vi "PID.vi"(1 "Present Value":dbl=15.0 format="%.2f", 2 "Previous Scan Value":dbl format="%.2f", 3 "Setpoint":dbl=15.0 format="%.2f") -> (0 "Dem Output":dbl format="%.2f")   [LabVIEW 2013]
uses:
  <vilib>/Analysis/NI_AALPro.lvlib
panel:
  in  "O/P deadband":dbl=1.0 format="%.2f"
  in  "Kp Deadband":dbl format="%.2f"
  in  "Derivative History":i32=20
  out "deadbanded error":dbl format="%.2f"
  in  "P":bool=TRUE
  in  "D":bool=TRUE
  in  "I":bool=TRUE
  out "Waveform Chart":T1(graph)
  in  "Manual Demand":dbl min=0.0 max=100.0 format="%.2f"
  in  "Manual Override":bool
  out "Control Sum":dbl format="%.2f"
  out "Derivative Term":dbl format="%.2f"
  out "Integral Term":dbl format="%.2f"
  out "error differential":dbl format="%.5f"
  out "error integral":dbl format="%.2f"
  out "Proportional Term":dbl format="%.2f"
  in  "Kd":dbl=25.0 format="%.2f"
  in  "Ki":dbl=0.03 format="%.3f"
  in  "Kp":dbl=1.5 format="%.2f"
  out "error":dbl format="%.2f"
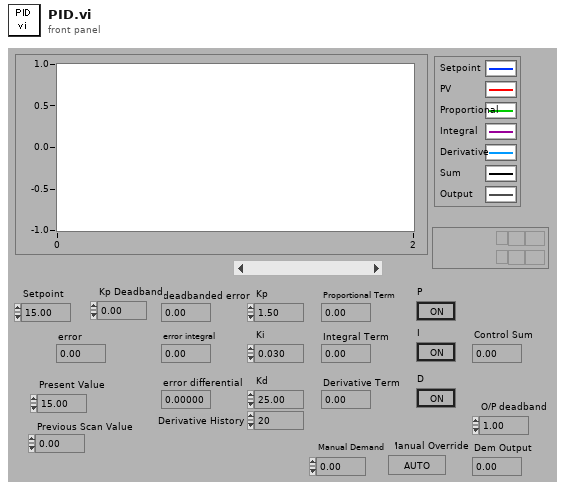
[diagram p1: front panel]
types:
  T1 = cluster{"Setpoint":dbl, "Present Value":dbl, "Proportional Term":dbl, "Integral Term":dbl, "Derivative Term":dbl, "Control Sum":dbl, "Dem Output":dbl}
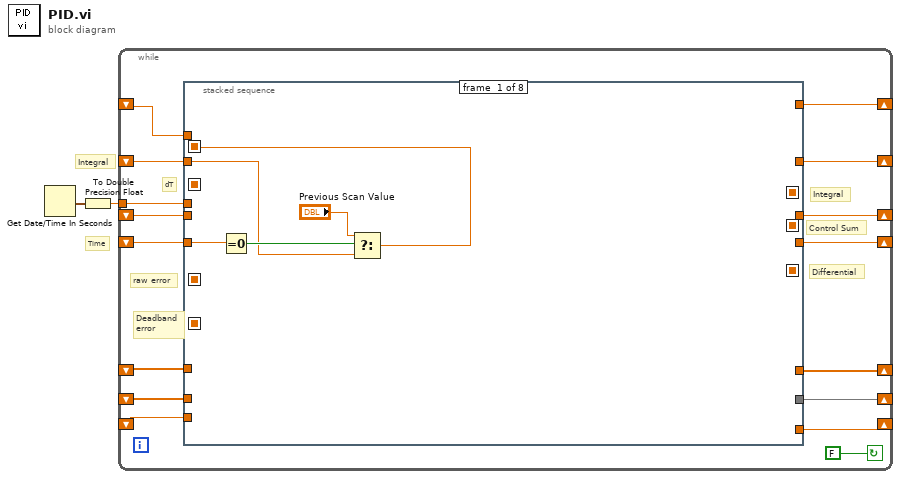
[diagram p0: block diagram]
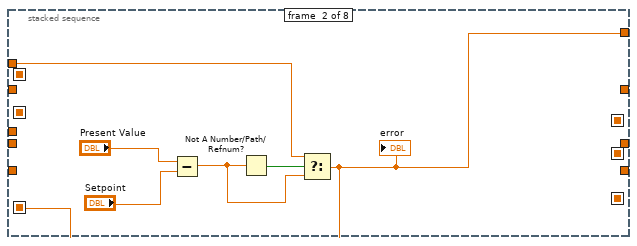
[diagram p2: hidden frame]
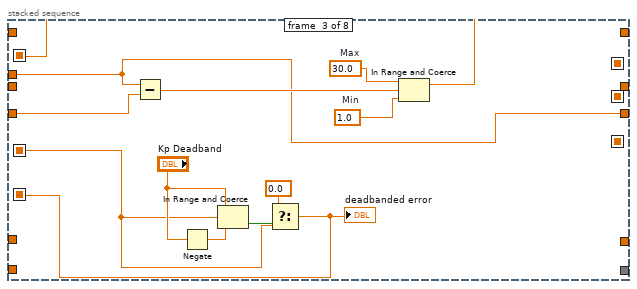
[diagram p3: hidden frame]
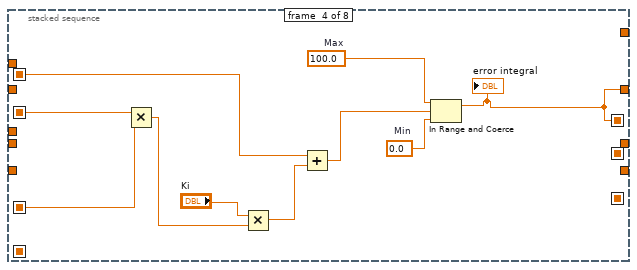
[diagram p4: hidden frame]
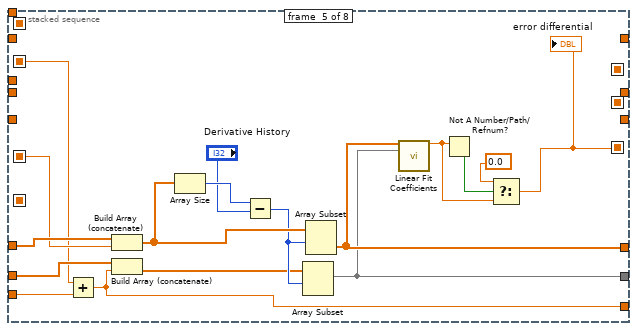
[diagram p5: hidden frame]
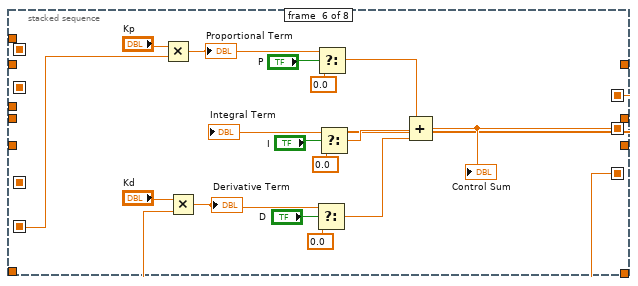
[diagram p6: hidden frame]
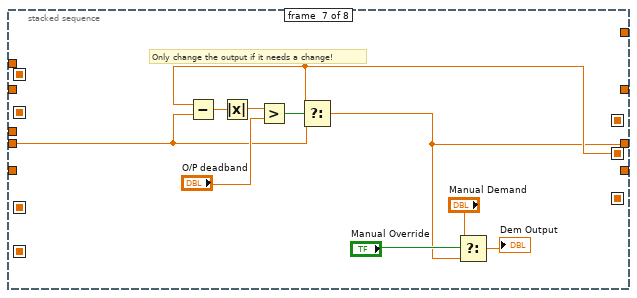
[diagram p7: hidden frame]
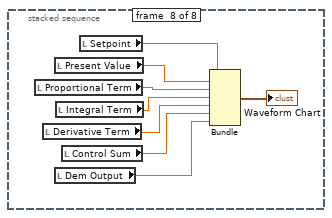
[diagram p8: hidden frame]
diagram:
  # "Integral"
  # "Time"
  n1 = Get Date/Time In Seconds() -> (seconds since 1Jan1904=w1:timestamp)
  n2 = To Double Precision Float(number=w1) -> (double precision float=w2:dbl)
  n3 = while {
    shift-left: _ -> [w5]
    shift-right: [w4] -> _
    shift-left: _ -> [w7]
    shift-right: [w6] -> _
    shift-left: _ -> [w9]
    shift-right: [w8] -> _
    tunnel: w2 -> [w14]
    shift-left: _ -> [w11]
    shift-right: [w10] -> _
    shift-left: _ -> [w13]
    shift-right: [w12] -> _
    shift-left: _ -> [w15]
    shift-right: [w16] -> _
    shift-left: _ -> [w18]
    shift-right: [w17] -> _
    stop <- FALSE continue-if-true
    # "Control Sum"
    # "raw error"
    # "Differential"
    # "Integral"
    # "Deadband\nerror"
    # "dT"
    n4 = stacked-sequence {
      seq-local: [_ _ w30 _ _ _ _ _] -> [_ _ _ w51 w54 _ _ _]
      seq-local: [_ _ w39 _ _ _ _ _] -> [_ _ _ _ _ w71 _ _]
      seq-local: [_ _ _ _ w59 _ _ _] -> [_ _ _ _ _ w70 _ _]
      seq-local: [_ _ _ w46 _ _ _ _] -> [_ _ _ _ _ w69 _ _]
      seq-local: [_ w24 _ _ _ _ _ _] -> [_ _ w31 w48 w60 _ _ _]
      seq-local: [_ _ _ _ _ w74 _ _] -> [_ _ _ _ _ _ w89 _]
      seq-local: [w19 _ _ _ _ _ _ _] -> [_ _ _ w42 _ _ _ _]
      tunnel: w18 -> [w23 _ w36 _ _ _ _ _]
      tunnel: [_ _ w34 _ _ _ _ _] -> w17
      tunnel: [_ _ _ w46 _ _ _ _] -> w16
      tunnel: w15 -> [w20 _ _ _ _ _ _ _]
      tunnel: w14 -> [_ _ w34 _ _ _ _ _]
      tunnel: w13 -> [_ _ _ _ w68 _ _ _]
      tunnel: [_ _ _ _ w61 _ _ _] -> w12
      tunnel: w11 -> [_ _ _ _ w67 _ _ _]
      tunnel: [_ _ _ _ w58 _ _ _] -> w10
      tunnel: w9 -> [_ _ _ _ _ _ w87 _]
      tunnel: [_ _ _ _ _ _ w86 _] -> w8
      tunnel: w7 -> [_ _ _ _ w53 _ _ _]
      tunnel: [_ _ _ _ w52 _ _ _] -> w6
      tunnel: w5 -> [_ w26 _ _ _ _ _ _]
      tunnel: [_ w24 _ _ _ _ _ _] -> w4
      frame #0 {
        n5 = Equal To 0?(x=w23) -> (x = 0?=w22:bool)
        n6 = Select(t="Previous Scan Value", s=w22, f=w20) -> (s? t:f=w19:dbl)
      }
      frame #1 {
        n7 = Subtract(x="Present Value", y="Setpoint") -> (x-y=w25:dbl)
        n8 = Not A Number/Path/Refnum?(number/path/refnum=w25) -> (NaN/Path/Refnum?=w27:bool)
        n9 = Select(t=w26, s=w27, f=w25) -> (s? t:f=w24:dbl)
        "error" <- w24
      }
      frame #2 {
        w37 = 1.0  # Min
        w38 = 30.0  # Max
        n10 = Subtract(x=w34, y=w36) -> (x-y=w35:dbl)
        n11 = Negate(x="Kp Deadband") -> (-x=w33:dbl)
        n12 = In Range and Coerce(upper limit="Kp Deadband", x=w31, lower limit=w33) -> (In Range?=w40:bool)  [unwired: 1 out]
        n13 = Select(t=0.0, s=w40, f=w31) -> (s? t:f=w39:dbl)
        "deadbanded error" <- w39
        n14 = In Range and Coerce(upper limit=w38, x=w35, lower limit=w37) -> (coerced(x)=w30:dbl)  [unwired: 1 out]
      }
      frame #3 {
        w50 = 0.0  # Min
        w45 = 100.0  # Max
        n15 = Multiply(x=w51, y=w48) -> (x*y=w44:dbl)
        n16 = Multiply(x="Ki", y=w44) -> (x*y=w47:dbl)
        n17 = Add(x=w42, y=w47) -> (x+y=w49:dbl)
        n18 = In Range and Coerce(upper limit=w45, x=w49, lower limit=w50) -> (coerced(x)=w46:dbl)  [unwired: 1 out]
        "error integral" <- w46
      }
      frame #4 {
        n19 = Add(x=w54, y=w53) -> (x+y=w52:dbl)
        n20 = Build Array (concatenate)(w68, w60) -> (w64:dbl[])
        n21 = Build Array (concatenate)(w67, w52) -> (w62:dbl[])
        n22 = Array Size(array=w64) -> (size(s)=w66:i32)
        n23 = Subtract(x=w66, y="Derivative History") -> (x-y=w63:i32)
        n24 = Array Subset(array=w62, index=w63) -> (w58:dbl[])  [unwired: 1 in]
        n25 = Array Subset(array=w64, index=w63) -> (w61:dbl[])  [unwired: 1 in]
        n26 = call <vilib>:"Linear Fit Coefficients.vi"("Y"=w61, "X"=w58) -> ("slope"=w55:dbl)  [unwired: 3 in, 10 out]
        n27 = Not A Number/Path/Refnum?(number/path/refnum=w55) -> (NaN/Path/Refnum?=w57:bool)
        n28 = Select(t=0.0 ("f"), s=w57, f=w55) -> (s? t:f=w59:dbl)
        "error differential" <- w59
      }
      frame #5 {
        n29 = Multiply(x="Kp", y=w71) -> (x*y=w83:dbl)
        "Proportional Term" <- w83
        n30 = Multiply(x="Kd", y=w70) -> (x*y=w75:dbl)
        "Derivative Term" <- w75
        n31 = Select(t=w75, s="D", f=0.0) -> (s? t:f=w77:dbl)
        n32 = Select(t=w83, s="P", f=0.0) -> (s? t:f=w84:dbl)
        n33 = Select(t=w69, s="I", f=0.0) -> (s? t:f=w76:dbl)
        n34 = Compound Arithmetic op=ADD(w84, w76, w77) -> (w74:dbl)
        "Control Sum" <- w74
        "Integral Term" <- w69
      }
      frame #6 {
        # "Only change the output if it needs a change!"
        n35 = Subtract(x=w89, y=w87) -> (x-y=w92:dbl)
        n36 = Absolute Value(x=w92) -> (abs(x)=w91:dbl)
        n37 = Greater?(x=w91, y="O/P deadband") -> (0:w90:bool)
        n38 = Select(t=w89, s=w90, f=w87) -> (s? t:f=w86:dbl)
        n39 = Select(t="Manual Demand", s="Manual Override", f=w86) -> (s? t:f=→"Dem Output":dbl)
      }
      frame #7 {
        n40 = local read "Proportional Term"() -> (w99:dbl)
        n41 = local read "Derivative Term"() -> (w101:dbl)
        n42 = local read "Present Value"() -> (w98:dbl)
        n43 = local read "Dem Output"() -> (w103:dbl)
        n44 = local read "Integral Term"() -> (w100:dbl)
        n45 = local read "Control Sum"() -> (w102:dbl)
        n46 = local read "Setpoint"() -> (w97:dbl)
        n47 = Bundle("Setpoint"=w97, "Present Value"=w98, "Proportional Term"=w99, "Integral Term"=w100, "Derivative Term"=w101, "Control Sum"=w102, "Dem Output"=w103) -> (→"Waveform Chart":T1)  [unwired: 1 out]
      }
    }
  }
